vi "Section Source.vi"(8 "Error In":errorcluster) -> (0 "Error Out":errorcluster)   [LabVIEW 2018, in "Tests.lvlib" / "Nodes.lvlib"]
uses:
  src/Toolkit/Low-Level/Nodes/Text/Text.lvclass
  D:/Users/cfield/Code/Field R&D Services/Mustache/trunk/src/Toolkit/Low-Level/Nodes/Abstract/Abstract.lvclass
  src/Toolkit/Low-Level/Nodes/Section/Section.lvclass
  Nodes.lvlib
  <vilib>/addons/_JKI Toolkits/Caraya/classes/Test/Test.lvclass
  <vilib>/addons/_JKI Toolkits/Caraya/classes/Assert/Assert.lvclass
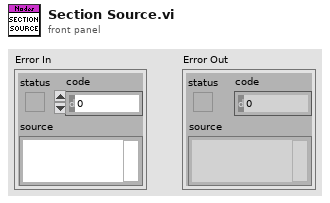
[diagram p1: front panel]
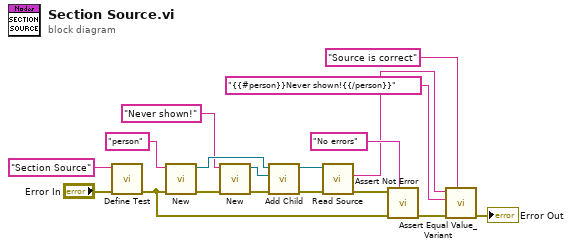
[diagram p0: block diagram]
diagram:
  n1 = call <vilib>:"Define Test.vi"("error in (no error)"="Error In", "Label (VI Title)"="Section Source") -> ("error out"=w10:errorcluster)  [unwired: 9 in]
  n2 = call "New.vi"("Error In"=w10, "Key"="person") -> ("Error Out"=w6:errorcluster, "Section"=w8:refnum<class "Section.lvclass">)  [unwired: 8 in]
  n3 = call "New.vi"("Error In"=w6, "Content"="Never shown!") -> ("Error Out"=w4:errorcluster, "Text"=w3:refnum<class "Text.lvclass">)  [unwired: 8 in]
  n4 = call-dynamic "Add Child.vi"("Error In"=w4, "Child"=w3, "Non-Terminal In"=w8) -> ("Error Out"=w2:errorcluster, "Non-Terminal Out"=w7:refnum<class "Section.lvclass">)  [unwired: 7 in]
  n5 = call-dynamic "Read Source.vi"("Error In"=w2, "Node In"=w7) -> ("Error Out"=w14:errorcluster, "Source"=w13:string)  [unwired: 7 in, 1 out]
  n6 = call <vilib>:"Assert Not Error.vi"("Label"="No errors", "error in (no error)"=w10, "Not Error?"=w14) -> ("error out"=w16:errorcluster)  [unwired: 8 in]
  n7 = call <vilib>:"Assert Equal Value_Variant.vi"("Label"="Source is correct", "error in (no error)"=w16, "Y"="{{#person}}Never shown!{{/person}}" ("format string"), "X"=w13) -> ("error out"=→"Error Out":errorcluster)  [unwired: 7 in]
